vi "Set Text File Sink Error.vi"(5 "Message Postfix":string, 7 "Error List":T1, 8 "error in (no error)":errorcluster, 11 "Text File Sink in":refnum<class "Text File Sink.lvclass">) -> (0 "error out":errorcluster, 3 "Text File Sink out":refnum<class "Text File Sink.lvclass">)   [LabVIEW 2016, in "Stream Log.lvlib" / "Text File Sink.lvclass"]
doc: "--\nCopyright © 2017 Composed SystemsI All rights reserved.\n\nAuthor: Jon McBee <jon.mcbee@composed.io>\n\nThis library is provided \"AS IS\" ,WITHOUT WARRANTIES OR\nCONDITIONS OF ANY KIND, either express or implied.\n\nComposed Systems -- composed.io\n\nStream 0.0.1.1\nJon McBee - Composed Systems\nCopyright (c) 2017, Composed Systems"
uses:
  <userlib>/Composed Systems/Stream/Log/Text File Sink/Text File Sink.lvclass
  C:/Program Files (x86)/National Instruments/LabVIEW 2016/user.lib/Composed Systems/Stream/Actor/Actor Class/Ancestral Actor.lvclass
  <userlib>/Composed Systems/Stream/Log/Text File Sink/Error List.ctl
  <userlib>/Composed Systems/Stream/Actor/Actor Class/Ancestral Actor.lvclass
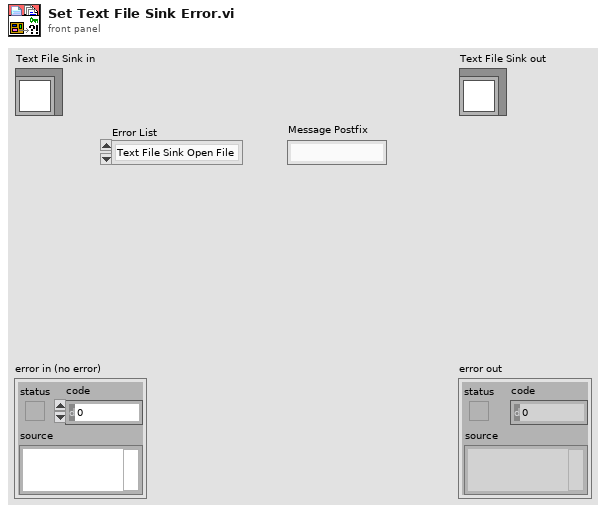
[diagram p1: front panel]
types:
  T1 = typedef "Stream Log.lvlib/Text File Sink.lvclass/Error List.ctl" = enum16{"Text File Sink Open File", "Add Header to Text File Sink", "Build Event Log Path"}
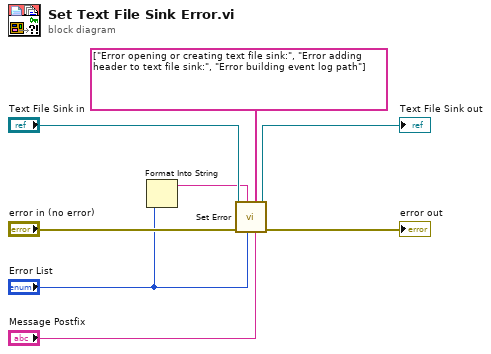
[diagram p0: block diagram]
diagram:
  n1 = Format Into String("Error List") -> (resulting string=w2:string)  [unwired: 3 in, 1 out]
  n2 = call <userlib>:"Set Error.vi"("Message Postfix"="Message Postfix", "Error Messages"=string[] ["Error opening or creating text file sink:", "Error adding header to text file sink:", "Error building event log path"], "Error Code"="Error List", "Error Name"=w2, "error in (no error)"="error in (no error)", "Actor in"="Text File Sink in") -> ("error out"=→"error out":errorcluster, "Actor out"=→"Text File Sink out":refnum<class "Text File Sink.lvclass">)  [unwired: 4 in]
